vi "1_CreateQueue.vi"(8 "error in (no error)":errorcluster caption="错误输入（无错误）", 11 "QueueName":T1) -> (0 "error out":errorcluster caption="错误输出", 3 "QueueOut":refnum<queue>[](array[refnum]))   [LabVIEW 2017]
uses:
  Ctrls/QueueDataForm.ctl
  Ctrls/QueueName.ctl
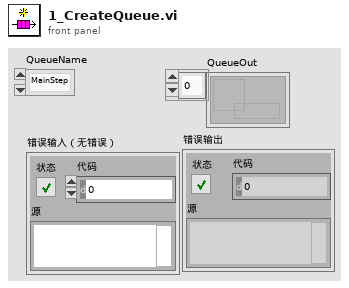
[diagram p1: front panel]
types:
  T1 = typedef "QueueName.ctl" = enum16{"MainStep", "AutoRun", "胶高"}
  T2 = typedef "QueueDataForm.ctl" = string
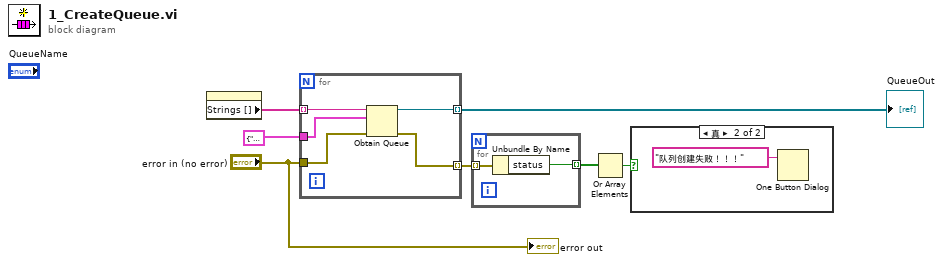
[diagram p0: block diagram]
diagram:
  n1 = property on="QueueName" class="Enum (严格)"() -> ("Strings []"=w7:string[])  [unwired: 2 in, 2 out]
  n2 = for {
    tunnel: w7 -> [w12] mode=indexing
    tunnel: cluster{"Cmd":T2, "Data":variant} {"Cmd"="", "Data"=variant} -> [w11]
    tunnel: [w10] -> w6 mode=indexing
    tunnel: "error in (no error)" -> [w9]
    tunnel: [w8] -> w5 mode=indexing
    n3 = Obtain Queue(name (unnamed)=w12, element data type=w11, error in (no error)=w9) -> (queue out=w10:refnum<queue>, error out=w8:errorcluster)  [unwired: 2 in, 1 out]
  }
  "QueueOut" <- w6
  n4 = for {
    tunnel: w5 -> [w14] mode=indexing
    tunnel: [w13] -> w4 mode=indexing
    n5 = Unbundle By Name(w14) -> ("status"=w13:bool)
  }
  n6 = Or Array Elements(Boolean array=w4) -> (logical OR=w3:bool)
  n7 = case shown="真" w3 {
    frame False {
    }
    frame True {
      n8 = One Button Dialog(message="队列创建失败！！！" ("消息")) -> ()  [unwired: 1 in, 1 out]
    }
  }
  "error out" <- "error in (no error)"
